vi "API get motor statue.vi"(11 "motor statue array input":i32[](array[numeric])) -> (1 "getmotorstatue return value":bool, 3 "motor statue array output":i32[](array[numeric]))   [LabVIEW 2011, in "API DYM.lvlib"]
uses:
  API DYM.lvlib
  DyMechnicalPlatform.dll
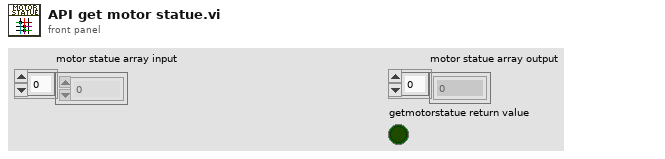
[diagram p1: front panel]
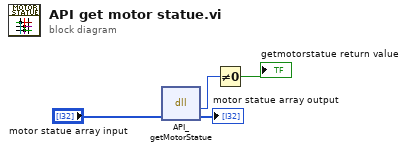
[diagram p0: block diagram]
diagram:
  n1 = dll-call lib="PTH1Xabs D可重构机电平台项目DemoLabViewDYSYSAPIDyMechnicalPlatform.dll" fn="API_getMotorStatue"("motor statue array"="motor statue array input") -> ("getmotorstatue return value"=w2:i32, "motor statue array"=→"motor statue array output":i32[])  [unwired: 3 in, 2 out]
  n2 = Not Equal To 0?(x=w2) -> (x != 0?=→"getmotorstatue return value":bool)
